vi "Config Type.vi"(11 "Start Seq Command in":refnum<class "Start Seq Command.lvclass">) -> (2 "Command Config Type":refnum<class "Command Config.lvclass">)   [LabVIEW 2020, in "VolatusSeq.lvlib" / "Start Seq Command.lvclass"]
uses:
  Start Seq Command.lvclass
  Start Seq Command.lvclass/Start Seq Command.ctl
  VolatusSeqConfig/Start Seq Command Config/Start Seq Command Config.lvclass
  C:/dev/lv20CE/relink/lv-volatus/VolatusSeqConfig/Command Config/Command Config.lvclass
  C:/dev/lv20CE/relink/lv-volatus/VolatusSeqConfig/Start Seq Command Config/Start Seq Command Config.lvclass
  VolatusSeqConfig/Command Config/Command Config.lvclass
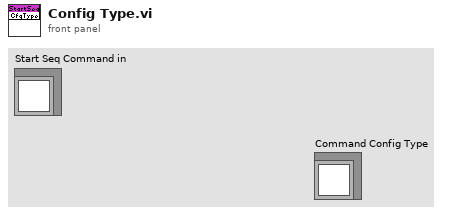
[diagram p1: front panel]
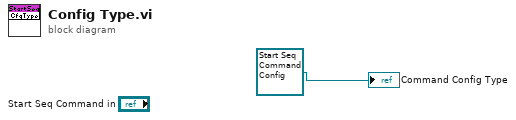
[diagram p0: block diagram]
diagram:
  "Command Config Type" <- refnum<class "Start Seq Command Config.lvclass"> refnum ("VolatusSeqConfig.lvlib:Start Seq Command Config.lvclass")
